vi "Key Generator.vi"(10 "error in (no error)":errorcluster, 11 "Bits (256)":i32=256) -> (2 "error out":errorcluster, 3 "Key":string)   [LabVIEW 2015, in "Crypto.lvlib"]
uses:
  Crypto.lvlib
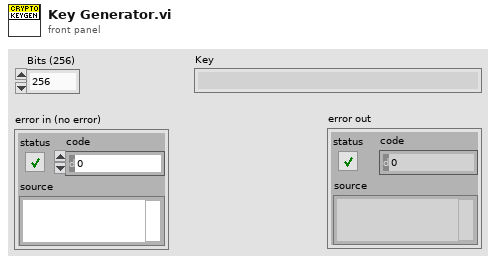
[diagram p1: front panel]
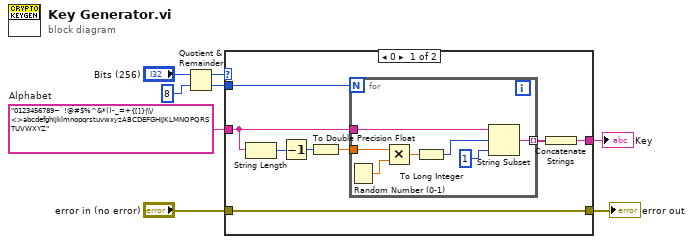
[diagram p0: block diagram]
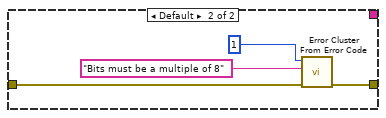
[diagram p2: hidden frame]
diagram:
  w4 = "0123456789~`!@#$%^&*()-_=+{[]}|\\/<>abcdefghijklmnopqrstuvwxyzABCDEFGHIJKLMNOPQRSTUVWXYZ"  # Alphabet
  n1 = Quotient & Remainder(x="Bits (256)", y=8) -> (x-y*floor(x/y)=w6:i32, floor(x/y)=w5:i32)
  n2 = case shown="0" w6 {
    tunnel: w5 -> [w16 _]
    tunnel: w4 -> [w15 _]
    tunnel: [w11 _] -> w3
    tunnel: "error in (no error)" -> [w10 w27]
    tunnel: [w10 w26] -> w1
    frame 0 {
      n3 = String Length(string=w15) -> (length=w14:i32)
      n4 = Decrement(x=w14) -> (x-1=w9:i32)
      n5 = To Double Precision Float(number=w9) -> (double precision float=w13:dbl)
      n6 = for {
        N: w16 -> [_]
        tunnel: w15 -> [w20]
        tunnel: w13 -> [w23]
        tunnel: [w17] -> w12 mode=indexing
        n7 = Random Number (0-1)() -> (number: 0 to 1=w22:dbl)
        n8 = Multiply(x=w23, y=w22) -> (x*y=w21:dbl)
        n9 = To Long Integer(number=w21) -> (32bit integer=w19:i32)
        n10 = String Subset(string=w20, offset (0)=w19, length (rest)=1 ("length (rest)")) -> (substring=w17:string)
      }
      n11 = Concatenate Strings(w12) -> (w11:string)
    }
    frame Default {
      n12 = call <vilib>:"Error Cluster From Error Code.vi"("error in (no error)"=w27, "error message (\"\")"="Bits must be a multiple of 8" ("error message (\"\")"), "error code (0)"=1) -> ("error out"=w26:errorcluster)  [unwired: 6 in]
    }
  }
  "Key" <- w3
  "error out" <- w1
